vi "PH_Cont-601k_PowerUnit.panel.vi"() -> ()   [LabVIEW 2014, in "PH_Cont-601k_PowerUnit.lvlib"]
uses:
  PH_Cont-601k_PowerUnit.lvlib
  PH_Cont-601k_PSU/PH_Cont-601k_PSU.Device Informaton.ctl
  PH_Cont-601k_PSU/PH_Cont-601k_PSU.Readyness.ctl
  PH_Cont-601k_PSU/PH_Cont-601k_PSU.Readyness Program.ctl
  PH_Cont-601k_PSU/PH_Cont-601k_PSU.Readyness Device.ctl
  PH_Cont-601k_PSU/PH_Cont-601k_PSU.Mode.ctl
  PH_Cont-601k_PSU/PH_Cont-601k_PSU.Configuration.ctl
  PH_Cont-601k_PSU/PH_Cont-601k_PSU.Device Status.ctl
  PH_StatusHandler/PH_StatusHandler.GUI element.ctl
  PH_PowerUnit_BaseClass/PH_PowerUnit_BaseClass.SM States.ctl
  PH_Cont-601k_PSU/PH_Cont-601k_PSU.GUI Refs.ctl
  PH_PowerUnit_BaseClass/PH_PowerUnit_BaseClass.GUI Refs to pack.ctl
  PH_PowerUnit_BaseClass/PH_PowerUnit_BaseClass.GUI Refs.ctl
  CSCore/CSObj/CSObj.lvlib
  CSCore/CSSystem/CSSystemLib/CSSystemLib.lvlib
  PH_Common/PH_Common.lvlib
  PH_Cont-601k_PSU/PH_Cont-601k_PSU.lvlib
  PH_PowerUnit_BaseClass/PH_PowerUnit_BaseClass.lvlib
  PH_Class/PH_Class.lvlib
  PH_StatusHandler/PH_StatusHandler.lvlib
panel:
  in  "Fire":bool
  out "Timeout SM":T1 caption="State PU"
  out "State SM":T1 caption="State PU"
  out "Waiting Time":dbl=999999.0
  out "Seq SM State":string
  out "PSDB Status":u32(colorbox)=6618880 caption="PSDB"
  in  "Tab Control":T2(tab)
  out "Interlock Indicator":u32(colorbox)=16860
  in  "Interlock":bool
  in  "Charge":bool
  in  "Mode":T3
  in  "Configuration":T4 items=["Ch intl, Fl intl, QSw intl", "Ch intl, Fl intl, QSw ext", "Ch intl, Fl ext, QSw intl", "Ch intl, Fl ext, QSw ext", "Ch ext, Fl int, QSw int", "Ch ext, Fl int, QSw ext", "Ch ext, Fl ext, QSw int", "Ch ext, Fl ext, QSw ext"]
  in  "Voltage":u16 caption="V" max=2000 step=10
  in  "Flash Interval":dbl caption="s" min=5.0 max=60.0 step=1.0
  out "Device Status":T5={"State"=0, "Interlocks"=[], "EOC"=16860, "Flashlamp Counter"=0, "error message"=""} {"State" items=["STOP: Stop Mode"=0, "STOP: Retrieve laser head serial number"=2, "STOP: Read flash and Q-switch counters"=3, "STOP: Keyswitch off"=5, "STOP: Delay for SmartBoard to get ready"=4, "STOP: SmartBoard download initialization"=6, "STOP: Retrieve SmartBoard version information"=7, "STOP: Retrieve all infos from SmartBoard"=8, "STOP: Stop Initialization"=10, "STOP: At Power-ON, found RUN, waiting for STOP"=15, "STOP: Idle, waiting for commands"=20, "STOP: Init laser head downloading process"=25, "STOP: Retrieve SmartBoard EEPROM location"=27, "STOP: Download laser head data"=30, "STOP: Initialize Power On Self Tests"=35, "STOP: Power On Self Test: Wait for pump to turn on"=40, "STOP: Power On Self Test: Wait for shutter to close"=45, "STOP: Power On Self Test: Wait for shutter to open"=50, "STANDBY: Standby Mode"=100, "STANDBY: Standby Initialization"=110, "STANDBY: Waiting for SmartBoard to complete a task"=113, "STANDBY: Idle, waiting for commands"=120, "STANDBY: Waiting for Smart Board to complete a task"=123, "STANDBY: At Power-ON, found READY. Waiting for STANDBY"=130, "READY: Ready Mode"=200, "READY: Ready Mode Initialization"=205, "READY: Begin Charging"=206, "READY: Wait for initial capacitor charge"=207, "READY: Charging"=208, "READY: Initial charge completion"=209, "READY: Idle, waiting for commands"=210, "READY: Uploading of paramters to the laser head"=215, "EMISSION: Emission Mode"=300, "EMISSION: Idle, waiting for commands"=310, "EMISSION: Waiting for shutter to close"=311, "EMISSION: Waiting to set pyro"=313, "EMISSION: Servo control to hold value"=315, "EMISSION: Servo context monitoring"=320, "EMISSION: Initialization for laser head pyro gein adjustment"=330, "EMISSION: Pyro gain adjustment - step 1"=335, "EMISSION: Pyro gain adjustment - step 2"=340, "EMISSION: Pyro gain adjustment - step 3"=345, "EMISSION: Pyro gain adjustment complete"=350, "ERROR: Error Mode"=400, "ERROR: Initialization for error mode"=405, "ERROR: Cooling Error - wating for STOP"=410, "ERROR: Error control for laser head not initialized fault."=415, "ERROR: Error control for TS-485 (Smart Bus) fault."=420, "ERROR: Error control for cover interlocks"=425, "ERROR: Watchdog Timeout"=435]}
  out "Power On":u32(colorbox)=16860
  in  "PU on":bool
  out "PSU On":u32(colorbox)=16860
  in  "Reset Error":bool
  in  "Expert working":bool
  out "Device Error":errorcluster caption="Error"
  out "Hard- and Software":T6={"VISA resource"="COM1", "Driver Revision"="", "Firmware Revision"=""}
  out "Readyness":T7
  out "Timing":u32(colorbox)=6618880
  out "Status":T10 caption="State PU"
  out "Chiller":u32(colorbox)=6618880
  in  "Exit":bool
  out "error out":errorcluster
  in  "Delete":bool
  in  "error in (no error)":errorcluster
  in  "object ref":refnum<vi>
  out "PreAmp":u32(colorbox)=6618880
  # "PCS"
  # "3.40"
  # "s"
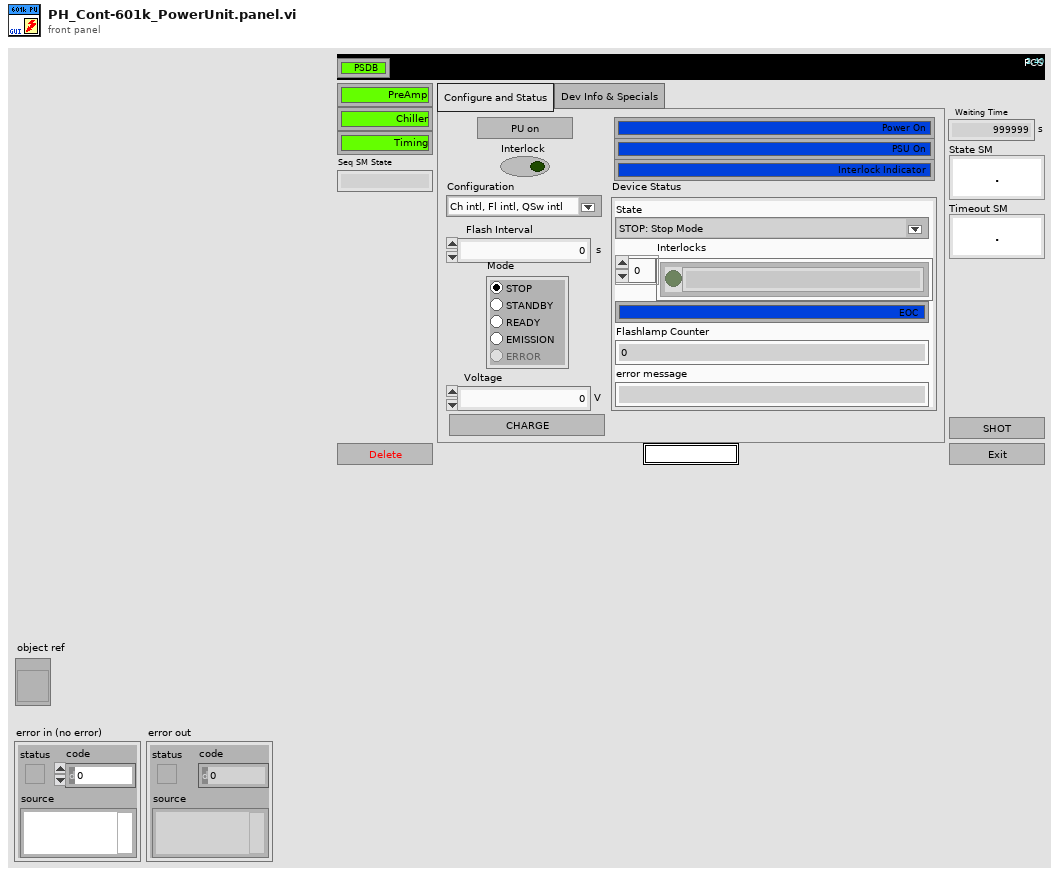
[diagram p1: front panel]
types:
  T1 = typedef "PH_PowerUnit_BaseClass.lvlib/PH_PowerUnit_BaseClass.SM States.ctl" = enum16{".", "Stand by", "Switch PU on", "Configure", "Set Default Voltage", "Set STANDBY", "Set READY", "Wait for Shot Cmd", "Open Dump Rods", "Open Ross Relais", "Close Ross Relais", "Switch PSU on", "Switch PSU off", "Charge", "Switch GD Channel on", "Close Dump Rods", "Rods-TO", "RR-TO", "PSU-TO", "Trigger-TO"}
  T2 = enum32{"Configure and Status", "Dev Info & Specials"}
  T3 = typedef "PH_Cont-601k_PSU.lvlib/PH_Cont-601k_PSU.Mode.ctl" = enum32{"STOP", "STANDBY", "READY", "EMISSION", "ERROR"}
  T4 = typedef "PH_Cont-601k_PSU.lvlib/PH_Cont-601k_PSU.Configuration.ctl" = u16
  T5 = typedef "PH_Cont-601k_PSU.lvlib/PH_Cont-601k_PSU.Device Status.ctl" = cluster{"State":u16, "Interlocks":cluster{"on/off":bool, "Explanation":string}[], "EOC":u32, "Flashlamp Counter":u32, "error message":string}
  T6 = typedef "PH_Cont-601k_PSU.lvlib/PH_Cont-601k_PSU.Device Informaton.ctl" = cluster{"VISA resource":refnum<visa-resource-name>, "Driver Revision":string, "Firmware Revision":string}
  T7 = typedef "PH_Cont-601k_PSU.lvlib/PH_Cont-601k_PSU.Readyness.ctl" = cluster{"Program":T8, "Device":T9}
  T8 = typedef "PH_Cont-601k_PSU.lvlib/PH_Cont-601k_PSU.Readyness Program.ctl" = enum32{"OFF", "POWER", "INTERLOCK"}
  T9 = typedef "PH_Cont-601k_PSU.lvlib/PH_Cont-601k_PSU.Readyness Device.ctl" = enum32{"OFF", "CONNECTING", "CONNECTED", "OPERATING", "EOC", "ERROR"}
  T10 = typedef "PH_StatusHandler.lvlib/PH_StatusHandler.GUI element.ctl" = u16
  T11 = typedef "PH_PowerUnit_BaseClass.lvlib/PH_PowerUnit_BaseClass.GUI Refs to pack.ctl" = cluster{"GUI Refs":T12, "Enabled":refnum<vi>, "PU on":refnum<vi>, "Waiting Time":refnum<vi>, "Timing.Instance":refnum<vi>, "Seq SM State":refnum<vi>, "Subscribed Trendmssgs":refnum<vi>[]}
  T12 = typedef "PH_PowerUnit_BaseClass.lvlib/PH_PowerUnit_BaseClass.GUI Refs.ctl" = cluster{"Delete Inst":refnum<vi>, "State TO SM":refnum<vi>, "State SM":refnum<vi>, "Fire":refnum<vi>}
  T13 = cluster{"GUI Refs Power Unit Base Class":T11, "PSDB Status":refnum<vi>}
  T14 = typedef "PH_Cont-601k_PSU.lvlib/PH_Cont-601k_PSU.GUI Refs.ctl" = cluster{"Power On":refnum<vi>, "Hard- and Software":refnum<vi>, "Device Status":refnum<vi>, "Device Error":refnum<vi>, "Configuration":refnum<vi>, "Flash Interval [s]":refnum<vi>, "Interlock":refnum<vi>, "Interlock Indicator":refnum<vi>, "Voltage [V]":refnum<vi>, "Readyness":refnum<vi>, "Mode":refnum<vi>, "Reset Error":refnum<vi>, "Expert working":refnum<vi>, "Charge":refnum<vi>, "PSU On":refnum<vi>}
  T15 = typedef "PH_Cont-601k_PSU.lvlib/PH_Cont-601k_PSU.i attribute.ctl" = cluster{"GUI Refs":T14, "Interlock":bool, "Service ID applied Voltage":i32, "Device Settings":cluster{"Configuration":T4, "Flash Interval [s]":dbl, "Mode":T3, "Voltage [V]":u16, "Charge":bool, "VISA resource name":refnum<visa-resource-name>}, "Readyness":T7, "Information":cluster{"VISA resource name":refnum<visa-resource-name>, "Tagname Power On":string, "Interlock":cluster{"Instance":string, "Tagname":string}, "Limits [V]":cluster{"Lower":dbl, "Upper":dbl}, "Tagname PSU On":string}, "R2S":bool, "Charge is allowed":bool}
  T16 = typedef "PH_PowerUnit_BaseClass.lvlib/PH_PowerUnit_BaseClass.i attribute.ctl" = cluster{"Constructor finished":bool, "PU":cluster{"In use":bool, "Service ID in use":i32, "GUI Ref":refnum<vi>}, "Enabling":cluster{"State":T17, "GUI Ref":refnum<vi>}, "Timing":cluster{"Last Shot":dbl, "Time between Shots [Sec]":dbl, "Waiting Time over?":bool, "Service ID Waiting Time":i32, "GUI Ref":refnum<vi>, "Instance":cluster{"Status":T18, "linked?":bool, "GUI Ref":refnum<vi>}}, "Sequencer":cluster{"SM State":string, "GUI Ref":refnum<vi>, "linked":bool}, "Subscribed Trendmssgs":cluster{"Tagname":string, "Status":T18, "linked?":bool, "Shot Condition":T18, "GUI Ref":refnum<vi>}[], "PP PU":T19, "Default Voltage (V)":dbl, "GUI Refs":T12, "PSDB data":cluster{"Shot Voltage [V]":dbl, "State TO SM":T1, "Write 2 early":bool}, "State TO SM":T1}
  T17 = typedef "PH_SystemInformation.lvlib/PH_SystemInformationEnabling State.ctl" = i32
  T18 = typedef "PH_StatusHandler.lvlib/PH_StatusHandler.Status.ctl" = i16
  T19 = typedef "PH_PP_Common.lvlib/PH_PP_Common.PUs.ctl" = enum16{"no Info", "PA-19mm-1", "PA-19mm-2", "PA-45mm-PILC", "PA-45mm-MAIN", "MA-PU-1", "MA-PU-2", "MA-PU-3", "MA-PU-4", "MA-PU-5", "MA-PU-6", "MA-FR", "MA-PILC", "PA-45mm-DP"}
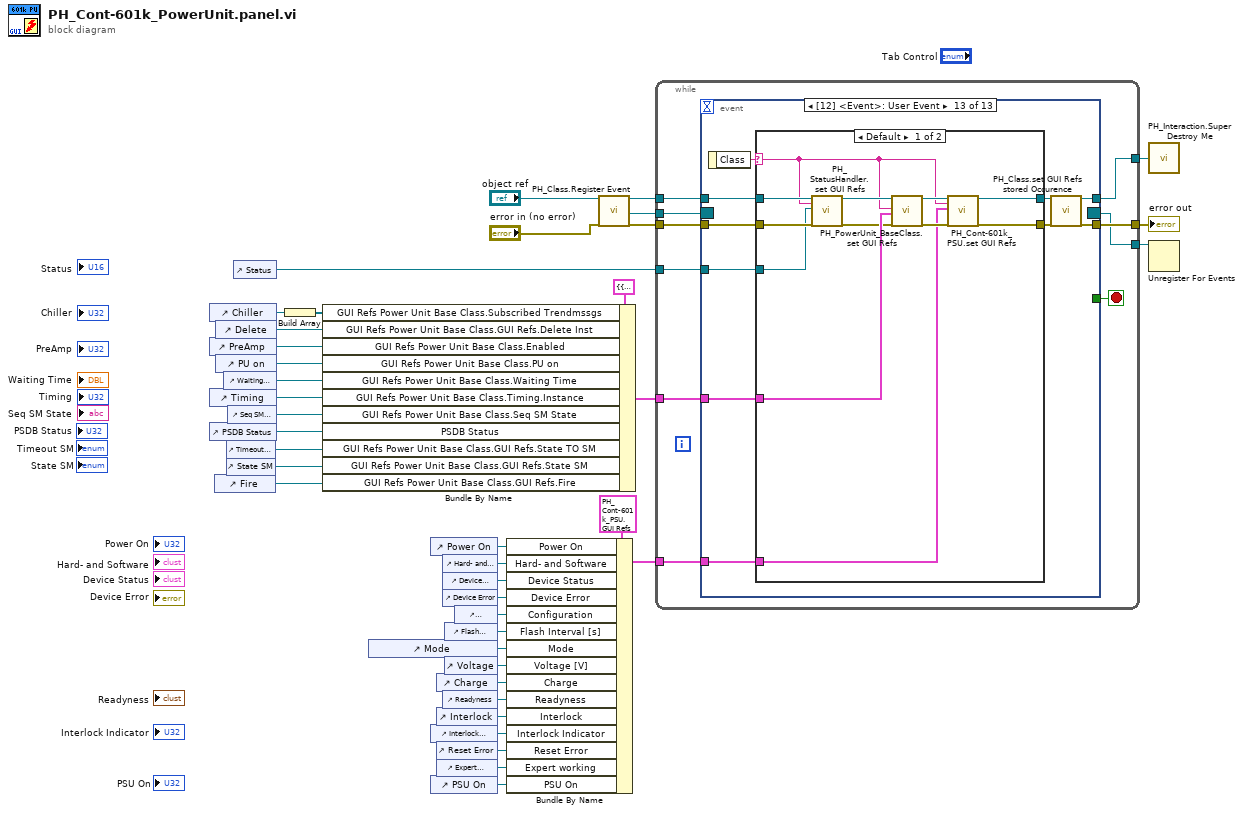
[diagram p0: block diagram]
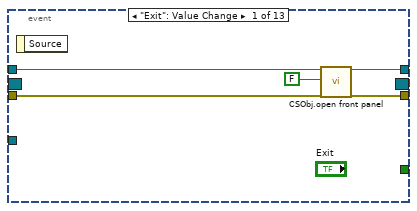
[diagram p2: hidden frame]
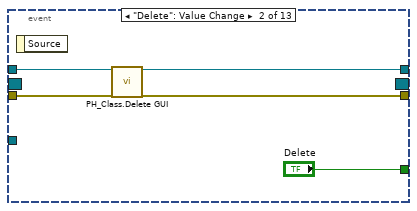
[diagram p3: hidden frame]
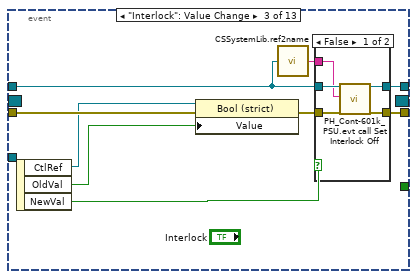
[diagram p4: hidden frame]
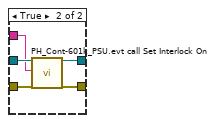
[diagram p5: hidden frame]
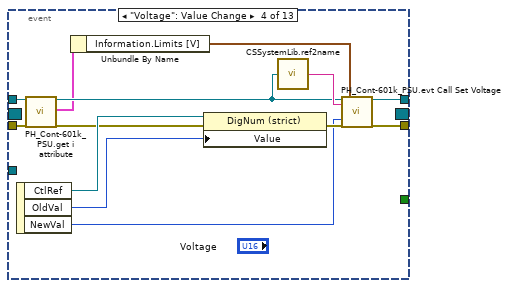
[diagram p6: hidden frame]
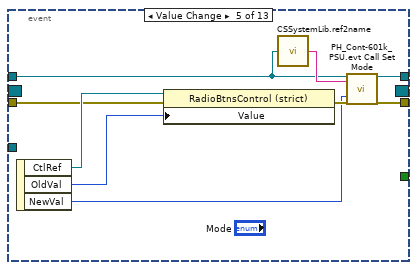
[diagram p7: hidden frame]
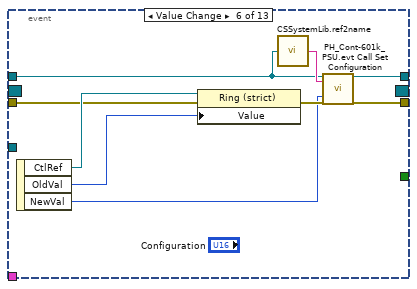
[diagram p8: hidden frame]
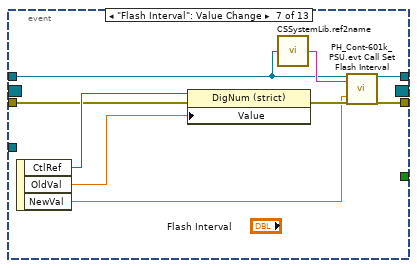
[diagram p9: hidden frame]
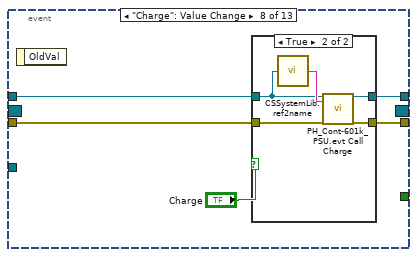
[diagram p10: hidden frame]
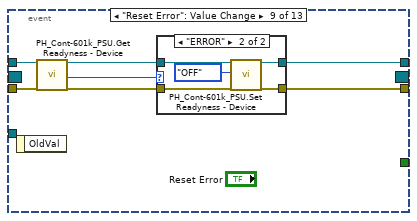
[diagram p12: hidden frame]
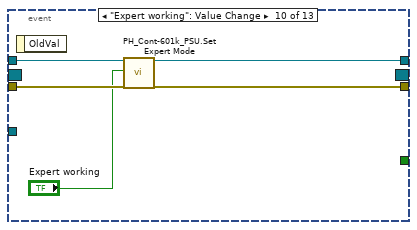
[diagram p14: hidden frame]
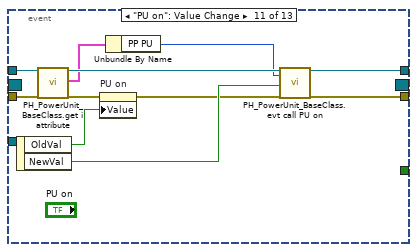
[diagram p15: hidden frame]
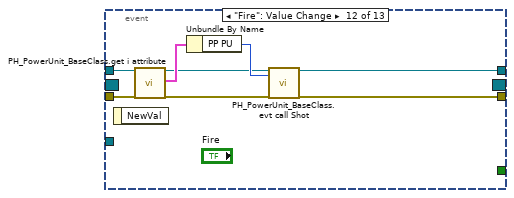
[diagram p16: hidden frame]
diagram:
  n1 = control-ref of="Chiller"() -> (w23:refnum<vi>)
  n2 = control-ref of="PreAmp"() -> (w15:refnum<vi>)
  n3 = control-ref of="Timing"() -> (w12:refnum<vi>)
  n4 = control-ref of="PSDB Status"() -> (w7:refnum<vi>)
  n5 = control-ref of="Fire"() -> (w4:refnum<vi>)
  n6 = control-ref of="Delete"() -> (w22:refnum<vi>)
  n7 = control-ref of="PU on"() -> (w14:refnum<vi>)
  n8 = control-ref of="Waiting Time"() -> (w13:refnum<vi>)
  n9 = control-ref of="Timeout SM"() -> (w2:refnum<vi>)
  n10 = control-ref of="State SM"() -> (w3:refnum<vi>)
  n11 = control-ref of="Seq SM State"() -> (w11:refnum<vi>)
  n12 = control-ref of="Status"() -> (w1:refnum<vi>)
  n13 = Build Array(w23) -> (w10:refnum<vi>[])
  n14 = Bundle By Name(cluster=T13 {"GUI Refs Power Unit Base Class"={"GUI Refs"={"Delete Inst"=refnum, "State TO SM"=refnum, "State SM"=refnum, "Fire"=refnum}, "Enabled"=refnum, "PU on"=refnum, "Waiting Time"=refnum, "Timing.Instance"=refnum, "Seq SM State"=refnum, "Subscribed Trendmssgs"=[]}, "PSDB Status"=refnum} ("GUI Refs"), "GUI Refs Power Unit Base Class.Subscribed Trendmssgs"=w10, "GUI Refs Power Unit Base Class.GUI Refs.Delete Inst"=w22, "GUI Refs Power Unit Base Class.Enabled"=w15, "GUI Refs Power Unit Base Class.PU on"=w14, "GUI Refs Power Unit Base Class.Waiting Time"=w13, "GUI Refs Power Unit Base Class.Timing.Instance"=w12, "GUI Refs Power Unit Base Class.Seq SM State"=w11, "PSDB Status"=w7, "GUI Refs Power Unit Base Class.GUI Refs.State TO SM"=w2, "GUI Refs Power Unit Base Class.GUI Refs.State SM"=w3, "GUI Refs Power Unit Base Class.GUI Refs.Fire"=w4) -> (w6:T13)
  n15 = control-ref of="Mode"() -> (w33:refnum<vi>)
  n16 = control-ref of="Power On"() -> (w39:refnum<vi>)
  n17 = control-ref of="Interlock Indicator"() -> (w28:refnum<vi>)
  n18 = control-ref of="PSU On"() -> (w5:refnum<vi>)
  n19 = control-ref of="Charge"() -> (w31:refnum<vi>)
  n20 = control-ref of="Interlock"() -> (w29:refnum<vi>)
  n21 = control-ref of="Reset Error"() -> (w27:refnum<vi>)
  n22 = control-ref of="Expert working"() -> (w26:refnum<vi>)
  n23 = control-ref of="Hard- and Software"() -> (w38:refnum<vi>)
  n24 = control-ref of="Device Status"() -> (w37:refnum<vi>)
  n25 = control-ref of="Device Error"() -> (w36:refnum<vi>)
  n26 = control-ref of="Readyness"() -> (w30:refnum<vi>)
  n27 = control-ref of="Flash Interval"() -> (w34:refnum<vi>)
  n28 = control-ref of="Voltage"() -> (w32:refnum<vi>)
  n29 = control-ref of="Configuration"() -> (w35:refnum<vi>)
  n30 = Bundle By Name(cluster=T14 {"Power On"=refnum, "Hard- and Software"=refnum, "Device Status"=refnum, "Device Error"=refnum, "Configuration"=refnum, "Flash Interval [s]"=refnum, "Interlock"=refnum, "Interlock Indicator"=refnum, "Voltage [V]"=refnum, "Readyness"=refnum, "Mode"=refnum, "Reset Error"=refnum, "Expert working"=refnum, "Charge"=refnum, "PSU On"=refnum} ("GUI Refs"), "Power On"=w39, "Hard- and Software"=w38, "Device Status"=w37, "Device Error"=w36, "Configuration"=w35, "Flash Interval [s]"=w34, "Mode"=w33, "Voltage [V]"=w32, "Charge"=w31, "Readyness"=w30, "Interlock"=w29, "Interlock Indicator"=w28, "Reset Error"=w27, "Expert working"=w26, "PSU On"=w5) -> (w17:T14)
  n31 = call "PH_Class.Register Event.vi"("i ref in"="object ref", "error in (no error)"="error in (no error)") -> ("i ref out"=w21:refnum<vi>, "Event Registration Refnum"=w19:refnum<event-registration>, "error out"=w20:errorcluster)  [unwired: 15 in]
  n32 = while {
    tunnel: w21 -> [w47]
    tunnel: [w46] -> w24
    tunnel: w20 -> [w49]
    tunnel: [w48] -> w25
    tunnel: w19 -> [w45]
    tunnel: [w44] -> w18
    tunnel: w17 -> [w43]
    tunnel: w6 -> [w42]
    tunnel: w1 -> [w41]
    stop <- w50 stop-if-true
    n33 = event shown="[12] <Event>: User Event" {
      selector: w45 -> [_ _ _ _ _ _ _ _ _ _ _ _ _]
      dyn-events: [_ _ _ _ _ _ _ _ _ _ _ _ _] -> w44
      timeout: _ -> [_ _ _ _ _ _ _ _ _ _ _ _ _]
      tunnel: [_ "Delete" _ _ _ _ _ _ _ _ _ _ _] -> w50
      tunnel: w47 -> [w52 w59 w66 w83 w94 w104 w112 w122 w136 w150 w154 w168 w177]
      tunnel: w49 -> [w55 w58 w63 w88 w93 w103 w111 w121 w135 w149 w158 w169 w175]
      tunnel: [w54 w56 w68 w91 w100 w109 w118 w123 w137 w147 w160 w162 w178] -> w48
      tunnel: [w51 w57 w69 w92 w101 w110 w119 w124 w138 w148 w159 w164 w179] -> w46
      tunnel: w43 -> [_ _ _ _ _ _ _ _ _ _ _ _ w172]
      tunnel: w42 -> [_ _ _ _ _ _ _ _ _ _ _ _ w171]
      tunnel: w41 -> [_ _ _ _ _ _ _ _ _ _ _ _ w170]
      event "Exit": Value Change {
        n34 = event-data() -> ()  [unwired: 1 in, 1 out]
        n35 = call "CSObj.open front panel.vi"("i ref in"=w52, "frontPanelOpen"=FALSE ("front panel open"), "error in (no error)"=w55) -> ("i ref out"=w51:refnum<vi>, "error out"=w54:errorcluster)  [unwired: 15 in]
      }
      event "Delete": Value Change {
        n36 = event-data() -> ()  [unwired: 1 in, 1 out]
        n37 = call "PH_Class.Delete GUI.vi"("VI in"=w59, "error in (no error)"=w58) -> ("VI out"=w57:refnum<vi>, "error out"=w56:errorcluster)  [unwired: 16 in]
      }
      event "Interlock": Value Change {
        n38 = event-data() -> ("CtlRef"=w62:refnum<vi>, "OldVal"=w61:bool, "NewVal"=w67:bool)  [unwired: 1 in]
        n39 = property class="Bool (strict)"(reference=w62, error in=w63, "Value"=w61) -> (error out=w64:errorcluster)  [unwired: 1 out]
        n40 = call "CSSystemLib.ref2name.vi"("obj refnum"=w66) -> ("name"=w65:string)
        n41 = case shown="False" w67 {
          tunnel: w66 -> [w74 w79]
          tunnel: w64 -> [w73 w78]
          tunnel: [w72 w77] -> w69
          tunnel: [w71 w76] -> w68
          tunnel: w65 -> [w70 w75]
          frame False {
            n42 = call "PH_Cont-601k_PSU.evt call Set Interlock Off.vi"("i ref in"=w74, "Instance name"=w70, "error in"=w73) -> ("i ref out"=w72:refnum<vi>, "error out"=w71:errorcluster)  [unwired: 15 in]
          }
          frame True {
            n43 = call "PH_Cont-601k_PSU.evt call Set Interlock On.vi"("i ref in"=w79, "Instance name"=w75, "error in"=w78) -> ("i ref out"=w77:refnum<vi>, "error out"=w76:errorcluster)  [unwired: 15 in]
          }
        }
      }
      event "Voltage": Value Change {
        n44 = event-data() -> ("CtlRef"=w87:refnum<vi>, "OldVal"=w86:u16, "NewVal"=w85:u16)  [unwired: 1 in]
        n45 = call "PH_Cont-601k_PSU.get i attribute.vi"("i ref in"=w83, "error in (no error)"=w88) -> ("i ref out"=w82:refnum<vi>, "i attribute"=w81:T15, "error out"=w84:errorcluster)  [unwired: 15 in]
        n46 = Unbundle By Name(w81) -> ("Information.Limits [V]"=w80:cluster{"Lower":dbl, "Upper":dbl})
        n47 = property class="DigNum (strict)"(reference=w87, error in=w84, "Value"=w86) -> (error out=w89:errorcluster)  [unwired: 1 out]
        n48 = call "CSSystemLib.ref2name.vi"("obj refnum"=w82) -> ("name"=w90:string)
        n49 = call "PH_Cont-601k_PSU.evt Call Set Voltage.vi"("i ref in"=w82, "Instance name"=w90, "Voltage to set [V]"=w85, "error in"=w89, "Limits [V]"=w80) -> ("i ref out"=w92:refnum<vi>, "error out"=w91:errorcluster)  [unwired: 13 in]
      }
      event Value Change {
        n50 = event-data() -> ("CtlRef"=w97:refnum<vi>, "OldVal"=w96:T3, "NewVal"=w95:T3)  [unwired: 1 in]
        n51 = property class="RadioBtnsControl (strict)"(reference=w97, error in=w93, "Value"=w96) -> (error out=w98:errorcluster)  [unwired: 1 out]
        n52 = call "CSSystemLib.ref2name.vi"("obj refnum"=w94) -> ("name"=w99:string)
        n53 = call "PH_Cont-601k_PSU.evt Call Set Mode.vi"("i ref in"=w94, "Instance name"=w99, "Mode to set"=w95, "error in"=w98) -> ("i ref out"=w101:refnum<vi>, "error out"=w100:errorcluster)  [unwired: 14 in]
      }
      event Value Change {
        n54 = event-data() -> ("CtlRef"=w106:refnum<vi>, "OldVal"=w105:T4, "NewVal"=w102:T4)  [unwired: 1 in]
        n55 = property class="Ring (strict)"(reference=w106, error in=w103, "Value"=w105) -> (error out=w107:errorcluster)  [unwired: 1 out]
        n56 = call "CSSystemLib.ref2name.vi"("obj refnum"=w104) -> ("name"=w108:string)
        n57 = call "PH_Cont-601k_PSU.evt Call Set Configuration.vi"("i ref in"=w104, "Instance name"=w108, "Configuration to set"=w102, "error in"=w107) -> ("i ref out"=w110:refnum<vi>, "error out"=w109:errorcluster)  [unwired: 14 in]
      }
      event "Flash Interval": Value Change {
        n58 = event-data() -> ("CtlRef"=w115:refnum<vi>, "OldVal"=w114:dbl, "NewVal"=w113:dbl)  [unwired: 1 in]
        n59 = property class="DigNum (strict)"(reference=w115, error in=w111, "Value"=w114) -> (error out=w116:errorcluster)  [unwired: 1 out]
        n60 = call "CSSystemLib.ref2name.vi"("obj refnum"=w112) -> ("name"=w117:string)
        n61 = call "PH_Cont-601k_PSU.evt Call Set Flash Interval.vi"("i ref in"=w112, "Instance name"=w117, "Flash Interval [s]"=w113, "error in"=w116) -> ("i ref out"=w119:refnum<vi>, "error out"=w118:errorcluster)  [unwired: 14 in]
      }
      event "Charge": Value Change {
        n62 = event-data() -> ()  [unwired: 1 in, 1 out]
        n63 = case shown="True" "Charge" {
          tunnel: [w126 w131] -> w124
          tunnel: [w125 w130] -> w123
          tunnel: w122 -> [w126 w128]
          tunnel: w121 -> [w125 w127]
          frame False {
          }
          frame True {
            n64 = call "CSSystemLib.ref2name.vi"("obj refnum"=w128) -> ("name"=w129:string)
            n65 = call "PH_Cont-601k_PSU.evt Call Charge.vi"("i ref in"=w128, "Instance name"=w129, "error in"=w127) -> ("i ref out"=w131:refnum<vi>, "error out"=w130:errorcluster)  [unwired: 15 in]
          }
        }
      }
      event "Reset Error": Value Change {
        n66 = event-data() -> ()  [unwired: 1 in, 1 out]
        n67 = call "PH_Cont-601k_PSU.Get Readyness - Device.vi"("VI in"=w136, "error in (no error)"=w135) -> ("VI out"=w134:refnum<vi>, "Readyness - Device"=w132:T9, "error out"=w133:errorcluster)  [unwired: 15 in]
        n68 = case shown="\"ERROR\"" w132 {
          tunnel: [w140 w145] -> w138
          tunnel: [w139 w144] -> w137
          tunnel: w134 -> [w140 w143]
          tunnel: w133 -> [w139 w142]
          frame Default {
          }
          frame "ERROR" {
            n69 = call "PH_Cont-601k_PSU.Set Readyness - Device.vi"("VI in"=w143, "Readyness - Device"=PH_Cont-601k_PSU.Readyness_Device."OFF", "error in (no error)"=w142) -> ("VI out"=w145:refnum<vi>, "error out"=w144:errorcluster)  [unwired: 15 in]
          }
        }
      }
      event "Expert working": Value Change {
        n70 = event-data() -> ()  [unwired: 1 in, 1 out]
        n71 = call "PH_Cont-601k_PSU.Set Expert Mode.vi"("VI in"=w150, "Expert working"="Expert working", "error in (no error)"=w149) -> ("VI out"=w148:refnum<vi>, "error out"=w147:errorcluster)  [unwired: 15 in]
      }
      event "PU on": Value Change {
        n72 = event-data() -> ("OldVal"=w156:bool, "NewVal"=w161:bool)  [unwired: 1 in]
        n73 = call "PH_PowerUnit_BaseClass.get i attribute.vi"("i ref in"=w154, "error in (no error)"=w158) -> ("i ref out"=w153:refnum<vi>, "i attribute"=w152:T16, "error out"=w155:errorcluster)  [unwired: 15 in]
        n74 = property on="PU on" class="Bool (strict)"(error in=w155, "Value"=w156) -> (error out=w157:errorcluster)  [unwired: 1 in, 1 out]
        n75 = Unbundle By Name(w152) -> ("PP PU"=w151:T19)
        n76 = call "PH_PowerUnit_BaseClass.evt call PU on.vi"("i ref in"=w153, "PowerUnit"=w151, "PU on"=w161, "error in (no error)"=w157) -> ("i ref out"=w159:refnum<vi>, "error out"=w160:errorcluster)  [unwired: 14 in]
      }
      event "Fire": Value Change {
        n77 = event-data() -> ()  [unwired: 1 in, 1 out]
        n78 = call "PH_PowerUnit_BaseClass.get i attribute.vi"("i ref in"=w168, "error in (no error)"=w169) -> ("i ref out"=w165:refnum<vi>, "i attribute"=w167:T16, "error out"=w163:errorcluster)  [unwired: 15 in]
        n79 = Unbundle By Name(w167) -> ("PP PU"=w166:T19)
        n80 = call "PH_PowerUnit_BaseClass.evt call Shot.vi"("i ref in"=w165, "PowerUnit"=w166, "error in (no error)"=w163) -> ("i ref out"=w164:refnum<vi>, "error out"=w162:errorcluster)  [unwired: 15 in]
      }
      event User Event {
        n81 = event-data() -> ("Class"=w173:string)  [unwired: 1 in]
        n82 = case shown="Default" w173 {
          selector: w173 -> [w181 _]
          tunnel: w177 -> [w183 w193]
          tunnel: [w188 w193] -> w176
          tunnel: w175 -> [w191 w192]
          tunnel: [w186 w192] -> w174
          tunnel: w172 -> [w185 _]
          tunnel: w171 -> [w190 _]
          tunnel: w170 -> [w180 _]
          frame Default {
            n83 = call "PH_StatusHandler.set GUI Refs.vi"("i ref in"=w183, "Class"=w181, "GUI Ref"=w180, "error in (no error)"=w191) -> ("i ref out"=w182:refnum<vi>, "error out"=w184:errorcluster)  [unwired: 14 in]
            n84 = call "PH_PowerUnit_BaseClass.set GUI Refs.vi"("i ref  in"=w182, "Class"=w181, "GUI Refs"=w190, "error in"=w184) -> ("i ref out"=w189:refnum<vi>, "error out"=w187:errorcluster)  [unwired: 14 in]
            n85 = call "PH_Cont-601k_PSU.set GUI Refs.vi"("VI in"=w189, "Class"=w181, "GUI Refs"=w185, "error in (no error)"=w187) -> ("VI out"=w188:refnum<vi>, "error out"=w186:errorcluster)  [unwired: 14 in]
          }
          frame "PH_Cont-601k_PowerUnit" {
          }
        }
        n86 = call "PH_Class.set GUI Refs stored Occurence.vi"("i ref in"=w176, "error in (no error)"=w174) -> ("i ref out"=w179:refnum<vi>, "error out"=w178:errorcluster)  [unwired: 16 in]
      }
    }
  }
  "error out" <- w25
  n87 = call "PH_Interaction.Super Destroy Me.vi"("i ref out"=w24) -> ()
  n88 = Unregister For Events(event registration refnum=w18) -> ()  [unwired: 1 in, 1 out]
